vi "Find and Rename VIs.vi"(0 "Owned Items[]":refnum<vi>[](array[refnum]), 5 "new name":string, 7 "name to replace":string, 11 "error in":errorcluster) -> (15 "error out":errorcluster)   [LabVIEW 2018, in "Springboard TLB`.lvlib"]
uses:
  Springboard TLB`.lvlib
  <vilib>/regexp/Match Regular Expression.xnode
panel:
  out "Array 2":string[](array[string])
  out "Array":string[](array[string])
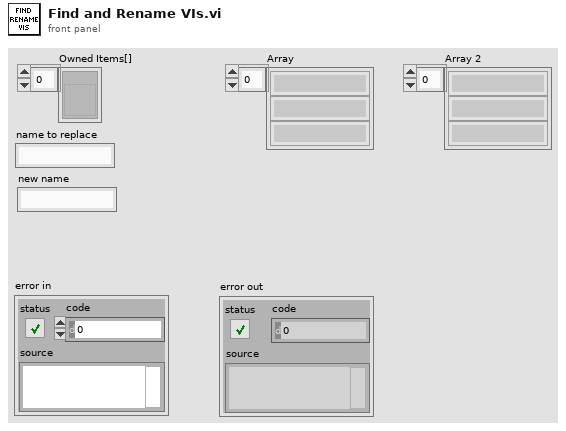
[diagram p1: front panel]
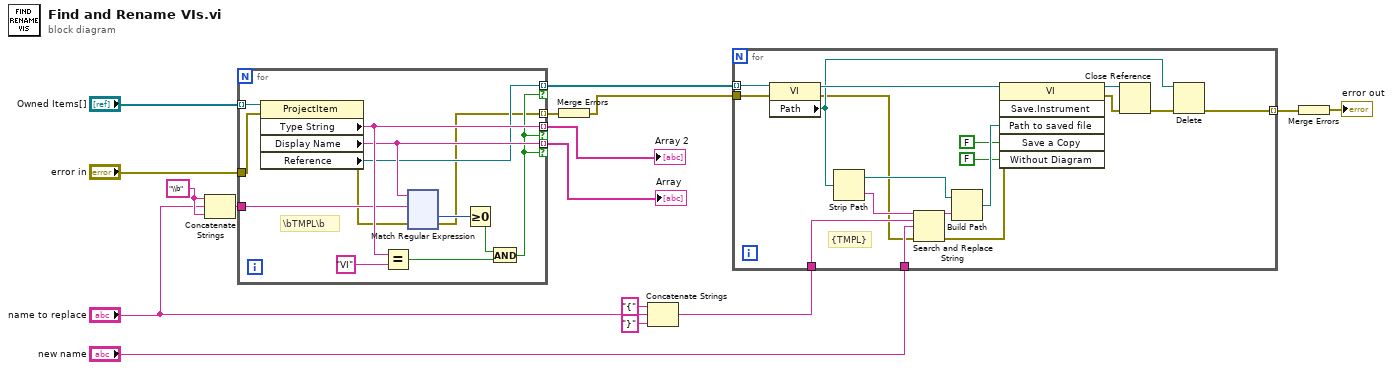
[diagram p0: block diagram]
diagram:
  w5 = "\\b" ("string")
  n1 = Concatenate Strings(w5, "name to replace", w5) -> (w6:string)
  n2 = for {
    tunnel: "Owned Items[]" -> [w29] mode=indexing
    tunnel: [w28] -> w10 mode=indexing if=w22
    tunnel: [w25] -> w11 mode=indexing if=w22
    tunnel: [w21] -> w14 mode=indexing if=w22
    tunnel: [w17] -> w15 mode=indexing
    tunnel: "error in" -> [w20]
    tunnel: w6 -> [w19]
    # "\\bTMPL\\b"
    n3 = property class="ProjectItem"(reference=w29, error in=w20) -> (error out=w18:errorcluster, "Type String"=w28:string, "Display Name"=w25:string, "Reference"=w21:refnum<vi>)  [unwired: 1 out]
    n4 = Equal?(x=w28, y="VI") -> (x = y?=w26:bool)
    n5 = xnode "Match Regular Expression"("input string"=w25, "regular expression"=w19, "error in"=w18) -> ("offset past match"=w24:i32, "error out"=w17:errorcluster)  [unwired: 3 in, 3 out]
    n6 = Greater Or Equal To 0?(x=w24) -> (x >= 0?=w23:bool)
    n7 = And(x=w23, y=w26) -> (x .and. y?=w22:bool)
  }
  "Array" <- w11
  "Array 2" <- w10
  n8 = Merge Errors(w15) -> (w16:errorcluster)
  n9 = Concatenate Strings("{" ("string"), "name to replace", "}" ("string")) -> (w1:string)
  n10 = for {
    tunnel: "new name" -> [w159]
    tunnel: w14 -> [w156] mode=indexing
    tunnel: w16 -> [w151]
    tunnel: [w148] -> w8 mode=indexing
    tunnel: w1 -> [w146]
    # "{TMPL}"
    n11 = property class="VI"(reference=w156, error in=w151) -> (reference out=w161:refnum<vi>, error out=w145:errorcluster, "Path"=w147:path)
    n12 = Strip Path(path=w147) -> (stripped path=w149:path, name=w160:string)
    n13 = Search and Replace String(input string=w160, search string=w146, replace string=w159, error in=w145) -> (result string=w158:string, error out=w144:errorcluster)  [unwired: 4 in, 2 out]
    n14 = Build Path(base path=w149, name or relative path=w158) -> (appended path=w157:path)
    n15 = invoke class="VI" method="Save.Instrument"(reference=w161, error in=w144, "Path to saved file"=w157, "Save a Copy"=FALSE, "Without Diagram"=FALSE) -> (reference out=w153:refnum<vi>, error out=w152:errorcluster)  [unwired: 1 in, 4 out]
    n16 = Close Reference(reference=w153, error in (no error)=w152) -> (error out=w150:errorcluster)
    n17 = Delete(path (use dialog)=w147, error in=w150) -> (error out=w148:errorcluster)  [unwired: 3 in, 2 out]
  }
  n18 = Merge Errors(w8) -> (→"error out":errorcluster)
